vi "Create 3D Steering Wheel from Params.vi"(5 "colors":T2={"wheel color"=4884736, "marker color"=590024}, 7 "dimensions":T1={"wheel thickness"=0.1, "axle radius"=0.05, "axle length"=0.025, "marker width"=0.005}, 8 "error in (no error)":errorcluster, 10 "wheel radius":dbl=0.25, 11 "name":string) -> (0 "error out":errorcluster, 1 "rotation axis":refnum<vi>, 2 "steering axis":refnum<vi>, 3 "3D steering wheel frame":refnum<vi>)   [LabVIEW 2017, in "NI_Robotics 3D Picture Steering Utilities.lvlib"]
doc: "Creates a 3D picture control mecanum wheel object."
uses:
  <vilib>/robotics/Steering/Utilities/3D Picture/NI_Robotics 3D Picture Steering Utilities.lvlib
  <vilib>/robotics/Steering/Utilities/3D Picture/Steering Wheel Colors.ctl
  <vilib>/robotics/Steering/Utilities/3D Picture/Steering Wheel Dimensions.ctl
  <vilib>/picture/3D Picture Control/Object/Create Object (name).vi
  <vilib>/picture/3D Picture Control/NI_3D Picture Control.lvlib
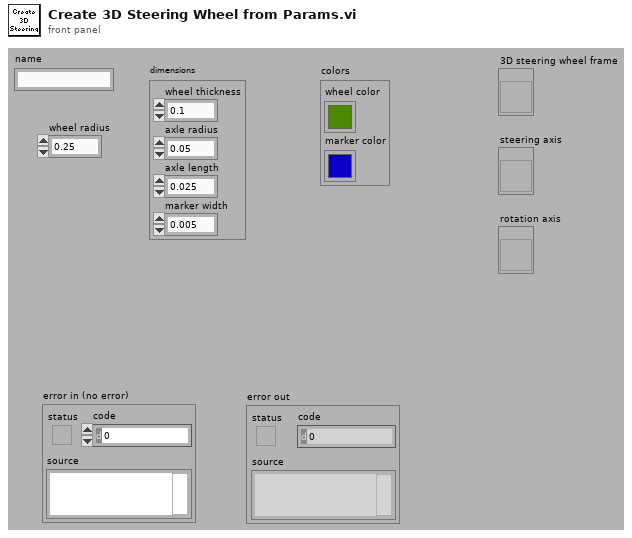
[diagram p1: front panel]
types:
  T1 = typedef "NI_Robotics 3D Picture Steering Utilities.lvlib/Steering Wheel Dimensions.ctl" = cluster{"wheel thickness":dbl, "axle radius":dbl, "axle length":dbl, "marker width":dbl}
  T2 = typedef "NI_Robotics 3D Picture Steering Utilities.lvlib/Steering Wheel Colors.ctl" = cluster{"wheel color":u32, "marker color":u32}
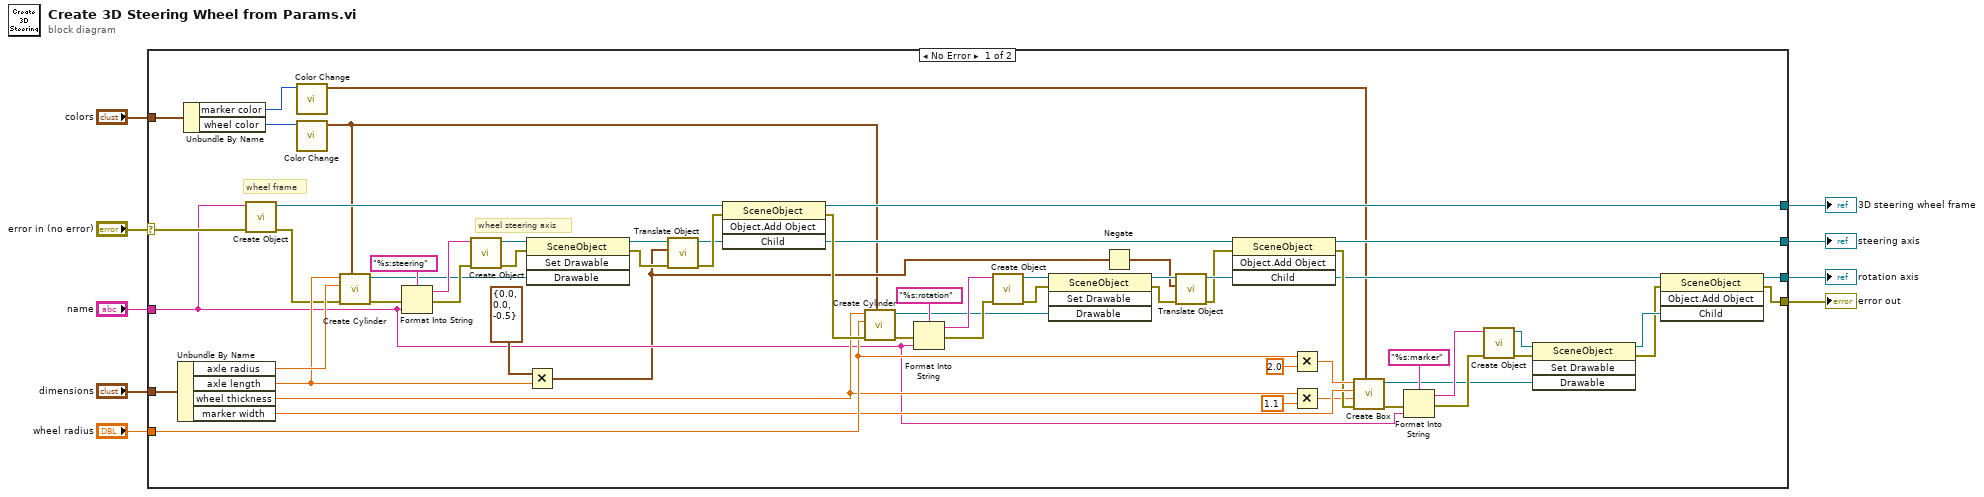
[diagram p0: block diagram]
diagram:
  n1 = case shown="No Error" "error in (no error)" {
    selector: "error in (no error)" -> [w53 w71]
    tunnel: [w55 _] -> w9
    tunnel: "dimensions" -> [w70 _]
    tunnel: "wheel radius" -> [w41 _]
    tunnel: "colors" -> [w69 _]
    tunnel: [w22 w71] -> w4
    tunnel: "name" -> [w21 _]
    tunnel: [w42 _] -> w2
    tunnel: [w25 _] -> w1
    frame No Error {
      # "wheel steering axis"
      # "wheel frame"
      n2 = Unbundle By Name(w70) -> ("axle radius"=w68:dbl, "axle length"=w61:dbl, "wheel thickness"=w35:dbl, "marker width"=w38:dbl)
      n3 = Unbundle By Name(w69) -> ("marker color"=w13:u32, "wheel color"=w11:u32)
      n4 = call-poly <vilib>:"Create Object.vi"("error in (no error)"=w53, "Name"=w21) -> ("error out"=w52:errorcluster, "Scene:New Object"=w54:refnum<vi>)  [unwired: 8 in]
      n5 = call <vilib>:"Color Change.vi"("Color"=w13) -> ("RGBA"=w12:cluster{"R":sgl, "G":sgl, "B":sgl, "A":sgl})  [unwired: 10 in]
      n6 = call <vilib>:"Color Change.vi"("Color"=w11) -> ("RGBA"=w10:cluster{"R":sgl, "G":sgl, "B":sgl, "A":sgl})  [unwired: 10 in]
      n7 = call <vilib>:"Create Cylinder.vi"("Color"=w10, "error in (no error)"=w52, "Radius"=w68, "Height"=w61) -> ("error out"=w59:errorcluster, "New Cylinder Refnum"=w20:refnum<vi>)  [unwired: 6 out]
      n8 = Format Into String(format string="%s:steering" ("Name"), error in=w59, w21) -> (resulting string=w56:string, error out=w58:errorcluster)  [unwired: 1 in]
      n9 = call-poly <vilib>:"Create Object.vi"("error in (no error)"=w58, "Name"=w56) -> ("error out"=w66:errorcluster, "Scene:New Object"=w67:refnum<vi>)  [unwired: 8 in]
      n10 = invoke class="SceneObject" method="Set Drawable"(reference=w67, error in=w66, "Drawable"=w20) -> (reference out=w63:refnum<vi>, error out=w65:errorcluster)  [unwired: 1 in, 2 out]
      n11 = Multiply(x=cluster{"X":sgl, "Y":sgl, "Z":sgl} {"X"=0.0, "Y"=0.0, "Z"=-0.5} ("Translation"), y=w61) -> (x*y=w15:cluster{"X":dbl, "Y":dbl, "Z":dbl})
      n12 = call <vilib>:"Translate Object.vi"("error in (no error)"=w65, "Translation"=w15, "Scene.Object In"=w63) -> ("error out"=w64:errorcluster, "Scene.Object Out"=w62:refnum<vi>)  [unwired: 7 out]
      n13 = invoke class="SceneObject" method="Object.Add Object"(reference=w54, error in=w64, "Child"=w62) -> (reference out=w55:refnum<vi>, error out=w51:errorcluster, "Child"=w43:refnum<vi>)  [unwired: 1 in, 1 out]
      n14 = call <vilib>:"Create Cylinder.vi"("Color"=w10, "error in (no error)"=w51, "Radius"=w41, "Height"=w35) -> ("error out"=w50:errorcluster, "New Cylinder Refnum"=w44:refnum<vi>)  [unwired: 6 out]
      n15 = Format Into String(format string="%s:rotation" ("Name"), error in=w50, w21) -> (resulting string=w47:string, error out=w48:errorcluster)  [unwired: 1 in]
      n16 = call-poly <vilib>:"Create Object.vi"("error in (no error)"=w48, "Name"=w47) -> ("error out"=w45:errorcluster, "Scene:New Object"=w46:refnum<vi>)  [unwired: 8 in]
      n17 = invoke class="SceneObject" method="Set Drawable"(reference=w46, error in=w45, "Drawable"=w44) -> (reference out=w19:refnum<vi>, error out=w17:errorcluster)  [unwired: 1 in, 2 out]
      n18 = Negate(x=w15) -> (-x=w14:cluster{"X":dbl, "Y":dbl, "Z":dbl})
      n19 = call <vilib>:"Translate Object.vi"("error in (no error)"=w17, "Translation"=w14, "Scene.Object In"=w19) -> ("error out"=w16:errorcluster, "Scene.Object Out"=w18:refnum<vi>)  [unwired: 7 out]
      n20 = invoke class="SceneObject" method="Object.Add Object"(reference=w43, error in=w16, "Child"=w18) -> (reference out=w42:refnum<vi>, error out=w37:errorcluster, "Child"=w26:refnum<vi>)  [unwired: 1 in, 1 out]
      n21 = Multiply(x=w41, y=2.0) -> (x*y=w39:dbl)
      n22 = Multiply(x=w35, y=1.1) -> (x*y=w34:dbl)
      n23 = call <vilib>:"Create Box.vi"("Color"=w12, "error in (no error)"=w37, "Length Z"=w34, "Length Y"=w38, "Length X"=w39) -> ("error out"=w33:errorcluster, "New Box Refnum"=w27:refnum<vi>)  [unwired: 5 in]
      n24 = Format Into String(format string="%s:marker" ("Name"), error in=w33, w21) -> (resulting string=w30:string, error out=w31:errorcluster)  [unwired: 1 in]
      n25 = call-poly <vilib>:"Create Object.vi"("error in (no error)"=w31, "Name"=w30) -> ("error out"=w28:errorcluster, "Scene:New Object"=w29:refnum<vi>)  [unwired: 8 in]
      n26 = invoke class="SceneObject" method="Set Drawable"(reference=w29, error in=w28, "Drawable"=w27) -> (reference out=w24:refnum<vi>, error out=w23:errorcluster)  [unwired: 1 in, 2 out]
      n27 = invoke class="SceneObject" method="Object.Add Object"(reference=w26, error in=w23, "Child"=w24) -> (reference out=w25:refnum<vi>, error out=w22:errorcluster)  [unwired: 1 in, 2 out]
    }
    frame Error {
    }
  }
  "3D steering wheel frame" <- w9
  "error out" <- w4
  "steering axis" <- w2
  "rotation axis" <- w1
